vi "volts to amp offset.vi"(10 "Low Volts":dbl, 11 "High Volts":dbl) -> (2 "DC Offset (0.00 V)":dbl, 3 "Amplitude (1.0 Vpp)":dbl)   [LabVIEW 2020]
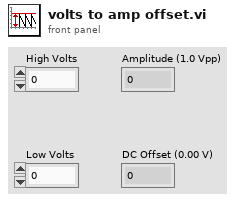
[diagram p1: front panel]
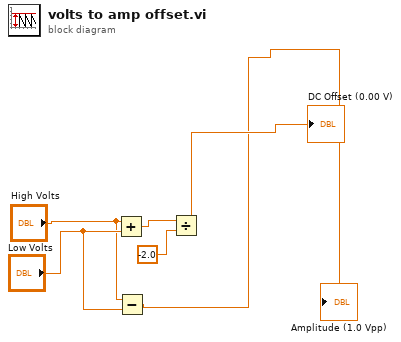
[diagram p0: block diagram]
diagram:
  n1 = Add(x="High Volts", y="Low Volts") -> (x+y=w2:dbl)
  n2 = Subtract(x="High Volts", y="Low Volts") -> (x-y=→"Amplitude (1.0 Vpp)":dbl)
  n3 = Divide(x=w2, y=-2.0) -> (x/y=→"DC Offset (0.00 V)":dbl)
